vi "Renishaw-XL80_GetEC10Status.vi"(8 "error in (no error)":errorcluster, 11 "Renishaw-XL80 in":refnum<class "Renishaw-XL80.lvclass">) -> (0 "error out":errorcluster, 2 "EC10Status":i32(ring) items=["EC10_CONNECTED"=0, "EC10_NOT_RESPONDING"=65536], 3 "Renishaw-XL80 out":refnum<class "Renishaw-XL80.lvclass">)   [LabVIEW 2024, in "Renishaw-XL80.lvclass"]
doc: "This read only property returns the current status of the EC10. It indicates whether or not the EC10 is responding.\n\nDefinition\nHRESULT\nget_EC10Status(\n [out, retval] EC10_STATUS_CODES* pVal\n);\n\nParameters\npVal\nA variable that will be set one of the EC10_STATUS_CODES.\n\nComments\nThis property will return with an HRESULT of E_FAIL if the client has not previously connected to a DX10 by calling Connect.\n\nThe property will normally return an HRESULT of S_OK. However, it will return E_POINTER if the client supplies a null pointer for pVal.\n\nNote: if there is a XL laser connected to the DX10Adaptor COM interface this property returns the status of the associated XC device"
uses:
  Renishaw-XL80.lvclass
  Renishaw-XL80.lvclass/Renishaw-XL80.ctl
  D:/A.C.M/Example CSharp_64/bin/Debug/Interop.DX10SDKADAPTORLib.dll
  Example CSharp_64/bin/Debug/Interop.DX10SDKADAPTORLib.dll
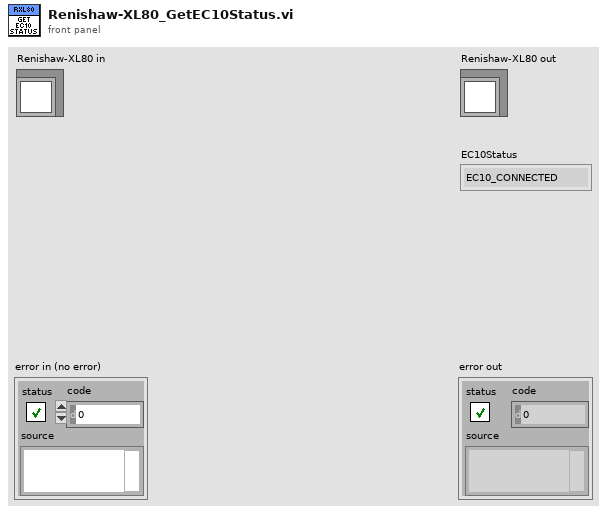
[diagram p1: front panel]
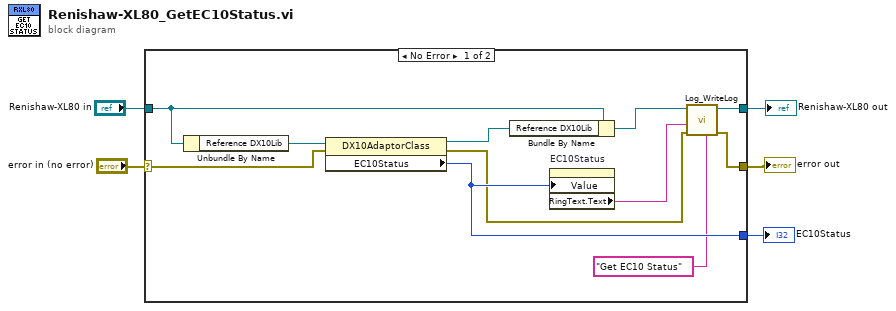
[diagram p0: block diagram]
diagram:
  n1 = case shown="No Error" "error in (no error)" {
    selector: "error in (no error)" -> [w13 w18]
    tunnel: [w8 w18] -> w4
    tunnel: [w10 w17] -> w2
    tunnel: "Renishaw-XL80 in" -> [w14 w17]
    tunnel: [w12 _] -> w1
    frame No Error {
      n2 = Unbundle By Name(w14) -> ("Reference DX10Lib"=w16:refnum<k24>)
      n3 = property class="DX10AdaptorClass"(reference=w16, error in=w13) -> (reference out=w15:refnum<k24>, error out=w6:errorcluster, "EC10Status"=w12:i32)
      n4 = Bundle By Name(cluster=w14, "Reference DX10Lib"=w15) -> (w11:refnum<class "Renishaw-XL80.lvclass">)
      n5 = property on="EC10Status" class="Ring (strict)"("Value"=w12) -> ("RingText.Text"=w9:string)  [unwired: 2 in, 2 out]
      n6 = call-dynamic "Log_WriteLog.vi"("Additional text"="Get EC10 Status", "error in (no error)"=w6, "Response"=w9, "Log in"=w11) -> ("error out"=w8:errorcluster, "Log out"=w10:refnum<class "Renishaw-XL80.lvclass">)  [unwired: 6 in]
    }
    frame Error {
    }
  }
  "error out" <- w4
  "Renishaw-XL80 out" <- w2
  "EC10Status" <- w1
